vi "Motors Move Constant Velocity.vi"(5 "Axis Multiplier":i32, 7 "Axis":i32, 8 "error in":errorcluster, 9 "VISA in":refnum<visa-resource-name>, 11 "Speed (mm/s)":dbl) -> (0 "error out":errorcluster, 1 "VISA out":refnum<visa-resource-name>)   [LabVIEW 2018]
panel:
  out "read buffer":string
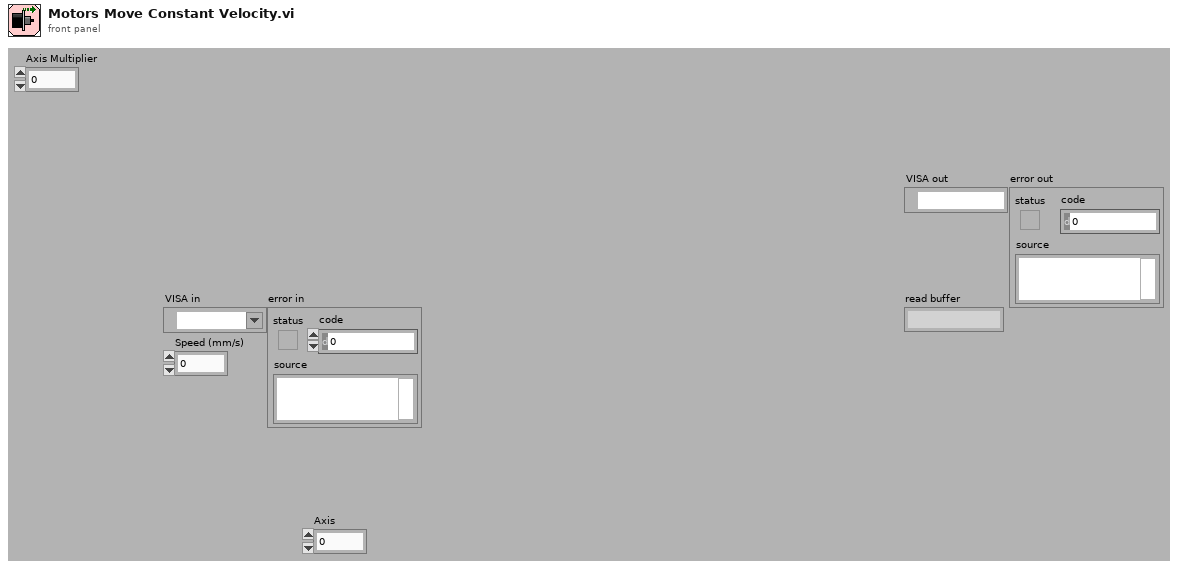
[diagram p1: front panel]
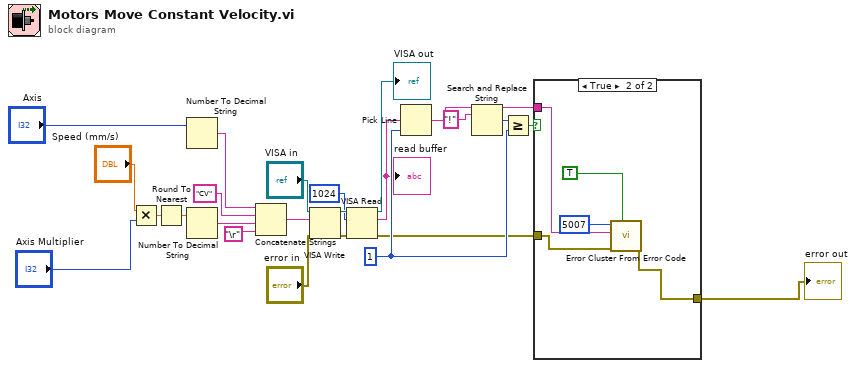
[diagram p0: block diagram]
diagram:
  w10 = 1 ("line index")
  n1 = Multiply(x="Speed (mm/s)", y="Axis Multiplier") -> (x*y=w15:dbl)
  n2 = Round To Nearest(number=w15) -> (nearest integer value=w4:dbl)
  n3 = Number To Decimal String(number="Axis") -> (decimal integer string=w23:string)  [unwired: 1 in]
  n4 = Number To Decimal String(number=w4) -> (decimal integer string=w14:string)  [unwired: 1 in]
  n5 = Concatenate Strings(w23, "CV" ("string"), w14, "\r") -> (w7:string)
  n6 = VISA Write(VISA resource name="VISA in", write buffer=w7, error in (no error)="error in") -> (VISA resource name out=w21:refnum<visa-resource-name>, error out=w20:errorcluster)  [unwired: 1 out]
  n7 = VISA Read(VISA resource name=w21, byte count=u32 1024, error in (no error)=w20) -> (VISA resource name out=→"VISA out":refnum<visa-resource-name>, read buffer=w6:string, error out=w1:errorcluster)  [unwired: 1 out]
  "read buffer" <- w6
  n8 = Pick Line(multi-line string=w6, line index=w10) -> (output string=w13:string)  [unwired: 1 in]
  n9 = Search and Replace String(input string=w13, search string="!" ("search string/char (-)")) -> (result string=w8:string, number of replacements=w11:i32)  [unwired: 6 in, 2 out]
  n10 = Greater Or Equal?(x=w11, y=w10) -> (x >= y?=w9:bool)
  n11 = case shown="True" w9 {
    tunnel: w8 -> [_ w28]
    tunnel: [w26 w30] -> w2
    tunnel: w1 -> [w26 w31]
    frame False {
    }
    frame True {
      n12 = call <vilib>:"Error Cluster From Error Code.vi"("show call chain? (False)"=TRUE, "error in (no error)"=w31, "error message (\"\")"=w28, "error code (0)"=5007) -> ("error out"=w30:errorcluster)  [unwired: 5 in]
    }
  }
  "error out" <- w2
